vi "setSerializedData.vi"(0 "reference":refnum<class "ClassNode.lvclass">, 1 "parent":refnum<class "AbstractNode.lvclass">, 2 "children":refnum<class "AbstractNode.lvclass">[](array[class]), 3 "xmlIn":string, 5 "error in (no error)":errorcluster) -> (14 "reference out":refnum<class "ClassNode.lvclass">, 19 "error out":errorcluster)   [LabVIEW 2014, in "ClassNode.lvclass"]
doc: "Sets stored data"
uses:
  <resource>/Framework/Providers/Open_GDS/UML/ClassNode_class/ClassNode.lvclass
  <resource>/Framework/Providers/Open_GDS/UML/AbstractNode_class/AbstractNode.lvclass
  <resource>/Framework/Providers/Open_GDS/UML/General/Rectangle/Rectangle Rectangle2D.ctl
  <resource>/Framework/Providers/Open_GDS/UML/MultiLineString_class/MultiLineString.lvclass
  <resource>/Framework/Providers/Open_GDS/UML/RectangularNode_class/RectangularNode.lvclass
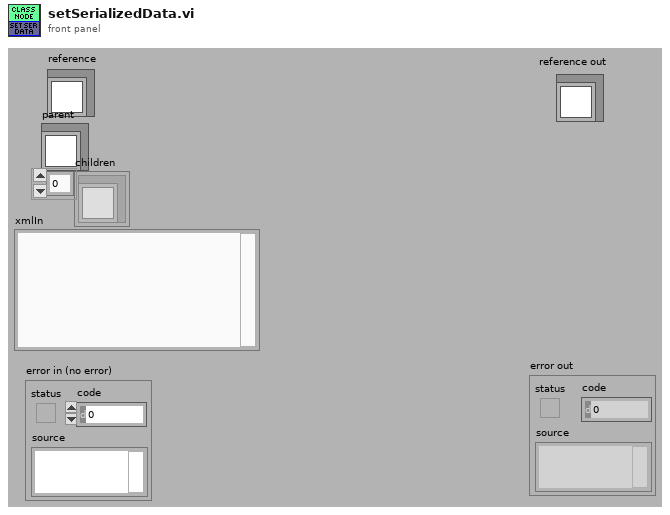
[diagram p1: front panel]
types:
  T1 = typedef "Rectangle Rectangle2D.ctl" = cluster{"x":dbl, "y":dbl, "width":dbl, "height":dbl}
  T2 = cluster{"Base class":cluster{"Base class":cluster{"parent":refnum<k1>, "children":refnum<k1>[], "Hidden":bool}, "bounds":T1}, "midHeight":dbl, "botHeight":dbl, "name":refnum<k1>, "attributes":refnum<k1>, "methods":refnum<k1>, "DEFAULT_COMPARTMENT_HEIGHT":i32, "DEFAULT_WIDTH":i32, "DEFAULT_HEIGHT":i32, "showMethods":bool, "showAttributes":bool, "ClassPath":path}
  T3 = cluster{"Attributes":cluster{"Base class":cluster{"Base class":cluster{"parent":refnum<k1>, "children":refnum<k1>[], "Hidden":bool}, "bounds":T1}, "midHeight":dbl, "botHeight":dbl, "name":refnum<k1>, "attributes":refnum<k1>, "methods":refnum<k1>, "DEFAULT_COMPARTMENT_HEIGHT":i32, "DEFAULT_WIDTH":i32, "DEFAULT_HEIGHT":i32, "showMethods":bool, "showAttributes":bool, "ClassPath":path}, string, string, string}
  T4 = typedef "ClassNode.lvclass/ObjectAttributes.ctl" = cluster{"midHeight":dbl, "botHeight":dbl, "name":refnum<class "MultiLineString.lvclass">, "attributes":refnum<class "MultiLineString.lvclass">, "methods":refnum<class "MultiLineString.lvclass">, "DEFAULT_COMPARTMENT_HEIGHT":i32, "DEFAULT_WIDTH":i32, "DEFAULT_HEIGHT":i32, "showMethods":bool, "showAttributes":bool, "ClassPath":path}
  T5 = typedef "RectangularNode.lvclass/ObjectAttributes.ctl" = cluster{"bounds":T1}
  T6 = typedef "AbstractNode.lvclass/ObjectAttributes.ctl" = cluster{"parent":refnum<class "AbstractNode.lvclass">, "children":refnum<class "AbstractNode.lvclass">[], "Hidden":bool}
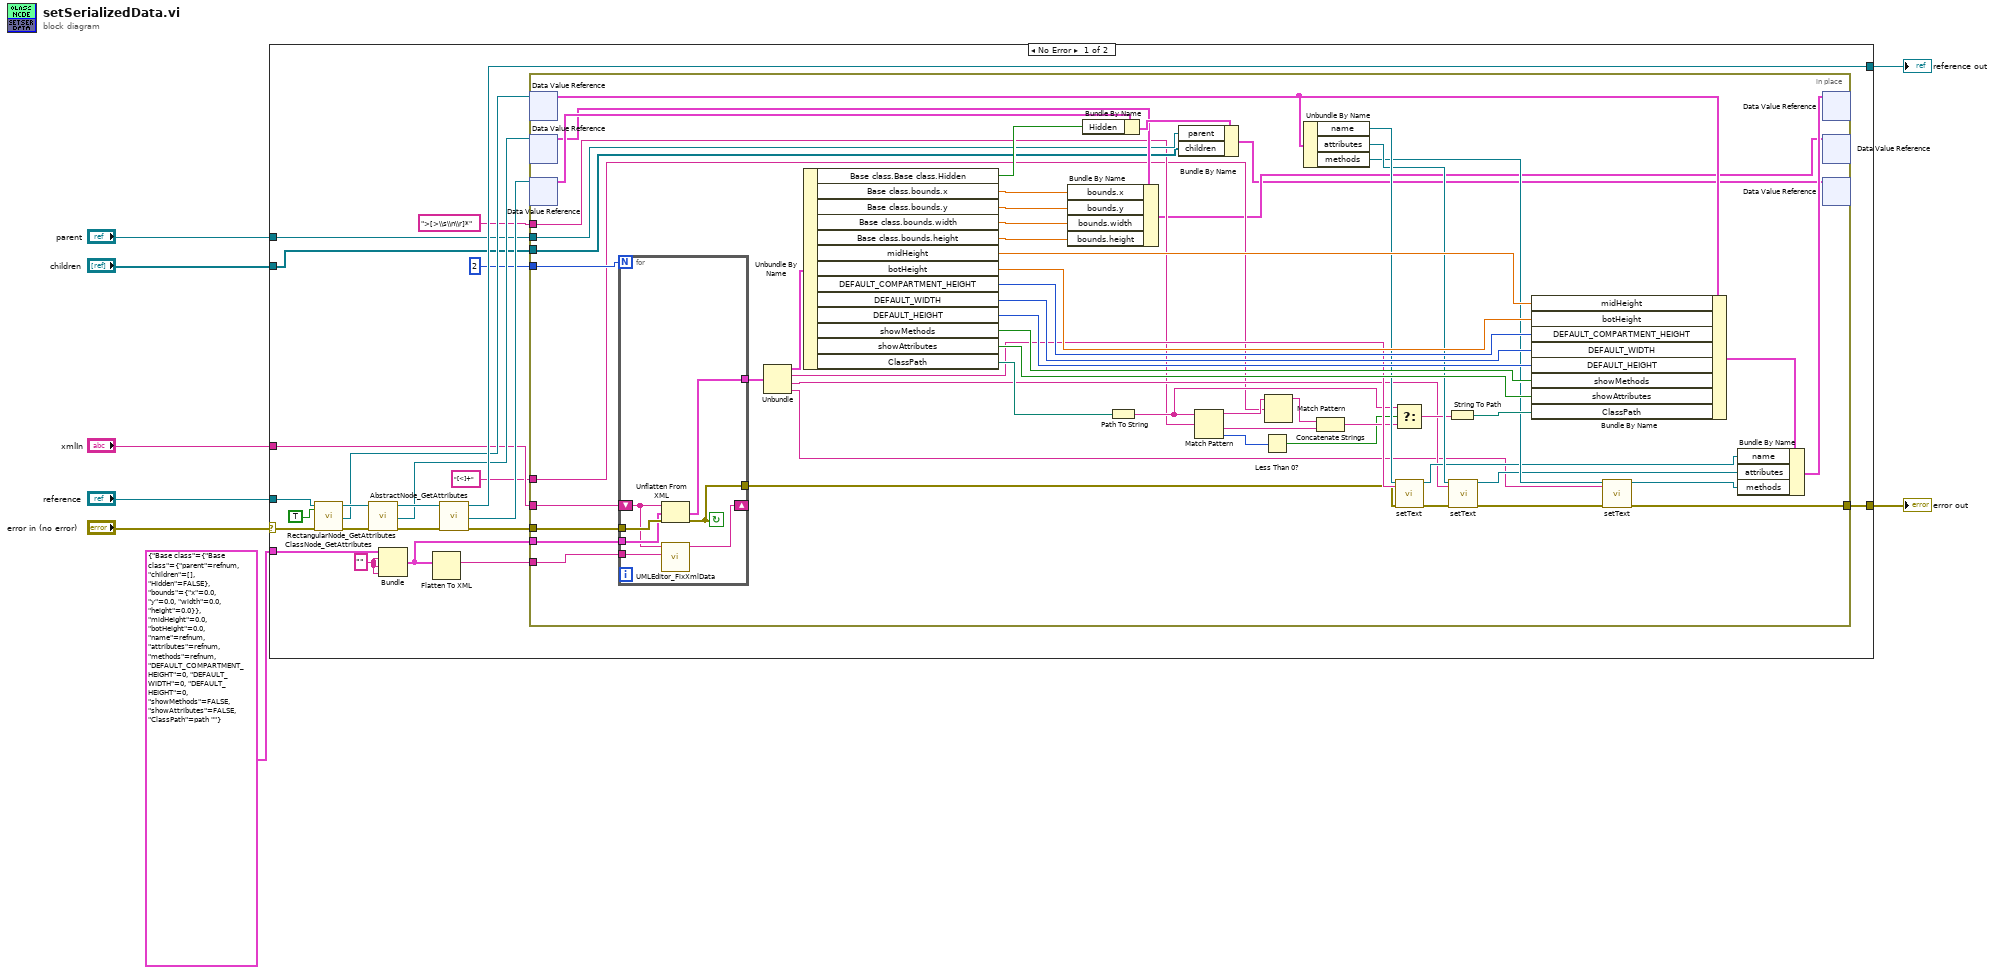
[diagram p0: block diagram]
diagram:
  n1 = case shown="No Error" "error in (no error)" {
    selector: "error in (no error)" -> [w29 w93]
    tunnel: "reference" -> [w30 w94]
    tunnel: [w28 w93] -> w6
    tunnel: [w31 w94] -> w5
    tunnel: "xmlIn" -> [w13 _]
    tunnel: "parent" -> [w12 _]
    tunnel: "children" -> [w11 _]
    tunnel: T2 {"Base class"={"Base class"={"parent"=refnum, "children"=[], "Hidden"=FALSE}, "bounds"={"x"=0.0, "y"=0.0, "width"=0.0, "height"=0.0}}, "midHeight"=0.0, "botHeight"=0.0, "name"=refnum, "attributes"=refnum, "methods"=refnum, "DEFAULT_COMPARTMENT_HEIGHT"=0, "DEFAULT_WIDTH"=0, "DEFAULT_HEIGHT"=0, "showMethods"=FALSE, "showAttributes"=FALSE, "ClassPath"=path ""} ("Attributes") -> [w26 _]
    frame No Error {
      w27 = ""
      n2 = call <resource>:"ClassNode_GetAttributes.vi"("reference in"=w30, "OnlyGetDvrReference(False)"=TRUE, "error in (no error)"=w29) -> ("reference out"=w24:refnum<class "ClassNode.lvclass">, "DataRef"=w20:refnum<data-value>, "error out"=w23:errorcluster)  [unwired: 13 in, 1 out]
      n3 = call <resource>:"RectangularNode_GetAttributes.vi"("reference in"=w24, "error in (no error)"=w23) -> ("reference out"=w22:refnum<class "ClassNode.lvclass">, "DataRef"=w19:refnum<data-value>, "error out"=w21:errorcluster)  [unwired: 14 in, 1 out]
      n4 = Bundle("Attributes"=w26, w27, w27, w27) -> (w14:T3)  [unwired: 1 out]
      n5 = Flatten To XML(anything=w14) -> (xml string=w15:string)
      n6 = call <resource>:"AbstractNode_GetAttributes.vi"("reference in"=w22, "error in (no error)"=w21) -> ("reference out"=w31:refnum<class "ClassNode.lvclass">, "DataRef"=w18:refnum<data-value>, "error out"=w16:errorcluster)  [unwired: 14 in, 1 out]
      n7 = in-place {
        in-place-border: [w54] -> w28
        in-place-border: 2 -> [w46]
        in-place-border: w16 -> [w45]
        in-place-border: w15 -> [w44]
        in-place-border: w14 -> [w43]
        in-place-border: w13 -> [w42]
        in-place-border: w12 -> [w41]
        in-place-border: w11 -> [w40]
        in-place-border: ">[>\\s\\n\\r]*" ("regular expression") -> [w39]
        in-place-border: "[<]+" ("regular expression") -> [w34]
        n8 = in-place-dvr #1(w20) -> (w85:T4)  [unwired: 1 out]
        n9 = in-place-dvr #2(w19) -> (w50:T5)  [unwired: 1 out]
        n10 = in-place-dvr #3(w18) -> (w52:T6)  [unwired: 1 out]
        n11 = for {
          N: w46 -> [_]
          tunnel: w45 -> [w92]
          tunnel: [w88] -> w59
          tunnel: [w91] -> w53
          tunnel: w44 -> [w90]
          tunnel: w43 -> [w89]
          shift-right: [w87] -> _
          shift-left: w42 -> [w86]
          stop <- w88 continue-if-true
          n12 = Unflatten From XML(xml string=w86, type=w89, error in (no error)=w92) -> (value=w91:T3, error out=w88:errorcluster)
          n13 = call <resource>:"UMLEditor_FixXmlData.vi"("XmlTemplateIn"=w90, "xmlIn"=w86) -> ("XML OUt"=w87:string)  [unwired: 9 in]
        }
        n14 = Unbundle(w53) -> ("Attributes"=w68:T2, w60:string, w57:string, w55:string)
        n15 = Unbundle By Name(w68) -> ("Base class.Base class.Hidden"=w67:bool, "Base class.bounds.x"=w66:dbl, "Base class.bounds.y"=w65:dbl, "Base class.bounds.width"=w64:dbl, "Base class.bounds.height"=w63:dbl, "midHeight"=w84:dbl, "botHeight"=w83:dbl, "DEFAULT_COMPARTMENT_HEIGHT"=w82:i32, "DEFAULT_WIDTH"=w81:i32, "DEFAULT_HEIGHT"=w80:i32, "showMethods"=w79:bool, "showAttributes"=w78:bool, "ClassPath"=w62:path)
        n16 = Bundle By Name(cluster=w50, "bounds.x"=w66, "bounds.y"=w65, "bounds.width"=w64, "bounds.height"=w63) -> (w33:T5)
        n17 = Bundle By Name(cluster=w52, "Hidden"=w67) -> (w51:T6)
        n18 = Path To String(path=w62) -> (string=w49:string)
        n19 = Bundle By Name(cluster=w51, "parent"=w41, "children"=w40) -> (w32:T6)
        n20 = Match Pattern(string=w49, regular expression=w39) -> (before substring=w38:string, after substring=w37:string, offset past match=w36:i32)  [unwired: 2 out]
        n21 = Less Than 0?(x=w36) -> (x < 0?=w47:bool)
        n22 = Match Pattern(string=w38, regular expression=w34) -> (before substring=w35:string)  [unwired: 4 out]
        n23 = Unbundle By Name(w85) -> ("name"=w75:refnum<class "MultiLineString.lvclass">, "attributes"=w74:refnum<class "MultiLineString.lvclass">, "methods"=w73:refnum<class "MultiLineString.lvclass">)
        n24 = Concatenate Strings(w35, w37) -> (w48:string)
        n25 = Select(t=w49, s=w47, f=w48) -> (s? t:f=w61:string)
        n26 = call-dynamic "setText.vi"("reference"=w75, "text"=w60, "error in (no error)"=w59) -> ("reference out"=w72:refnum<class "MultiLineString.lvclass">, "error out"=w58:errorcluster)  [unwired: 15 out]
        n27 = String To Path(string=w61) -> (path=w77:path)
        n28 = call-dynamic "setText.vi"("reference"=w74, "text"=w57, "error in (no error)"=w58) -> ("reference out"=w71:refnum<class "MultiLineString.lvclass">, "error out"=w56:errorcluster)  [unwired: 15 out]
        n29 = Bundle By Name(cluster=w85, "midHeight"=w84, "botHeight"=w83, "DEFAULT_COMPARTMENT_HEIGHT"=w82, "DEFAULT_WIDTH"=w81, "DEFAULT_HEIGHT"=w80, "showMethods"=w79, "showAttributes"=w78, "ClassPath"=w77) -> (w76:T4)
        n30 = call-dynamic "setText.vi"("reference"=w73, "text"=w55, "error in (no error)"=w56) -> ("reference out"=w70:refnum<class "MultiLineString.lvclass">, "error out"=w54:errorcluster)  [unwired: 15 out]
        n31 = Bundle By Name(cluster=w76, "name"=w72, "attributes"=w71, "methods"=w70) -> (w69:T4)
        n32 = in-place-dvr #1(w69) -> ()  [unwired: 2 out]
        n33 = in-place-dvr #2(w33) -> ()  [unwired: 2 out]
        n34 = in-place-dvr #3(w32) -> ()  [unwired: 2 out]
      }
    }
    frame Error {
    }
  }
  "reference out" <- w5
  "error out" <- w6
